vi "power.vi"(0 "Channel Index":i32, 5 "Clear PCM Sticky Faults":bool, 7 "Tare PDP Currents":bool, 9 "Clear PDP Sticky Faults":bool, 11 "Reset PDP Energy":bool) -> (4 "roboRIO":T4, 6 "Rail Voltages":T3, 8 "PCM":T2, 10 "PDP":T1, 13 "Channel Content":string, 15 "OutputsEnabled?":bool)   [LabVIEW 2014]
uses:
  Type Defs/power data.ctl
  <vilib>/Rock Robotics/Network Tables/NT Read String Array.vi
  <vilib>/Rock Robotics/Network Tables/NT Write Boolean Array.vi
  <vilib>/Rock Robotics/Network Tables/NT Read Boolean Array.vi
  <vilib>/Rock Robotics/Network Tables/NT Read Numeric Array.vi
  <vilib>/Rock Robotics/Network Tables/NT Read String.vi
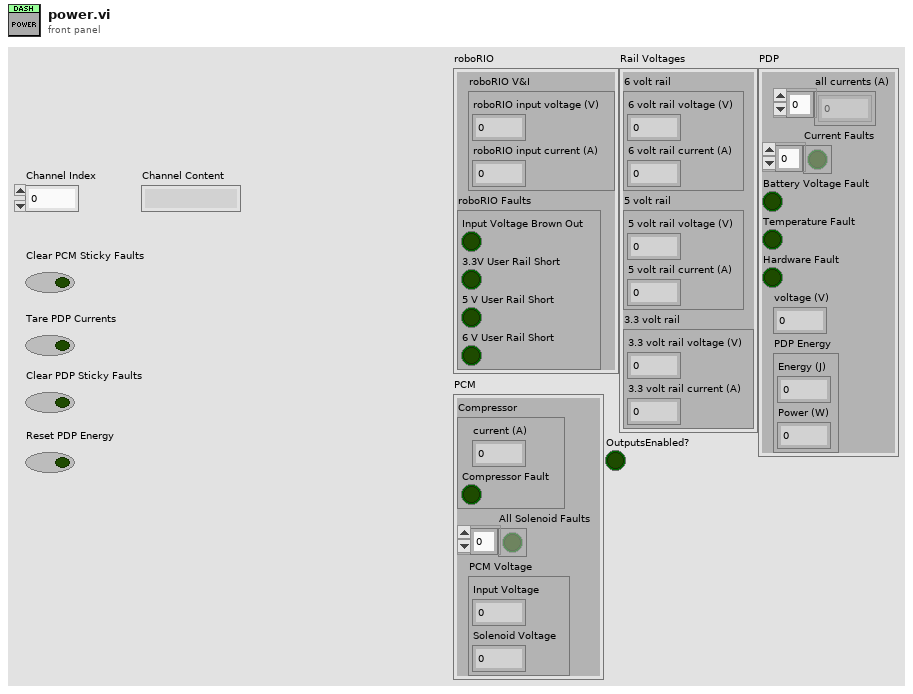
[diagram p1: front panel]
types:
  T1 = cluster{"all currents (A)":dbl[], "Current Faults":bool[], "Battery Voltage Fault":bool, "Temperature Fault":bool, "Hardware Fault":bool, "voltage (V)":dbl, "PDP Energy":cluster{"Energy (J)":dbl, "Power (W)":dbl}}
  T2 = cluster{"Compressor":cluster{"current (A)":dbl, "Compressor Fault":bool}, "All Solenoid Faults":bool[], "PCM Voltage":cluster{"Input Voltage":dbl, "Solenoid Voltage":dbl}}
  T3 = cluster{"6 volt rail":cluster{"6 volt rail voltage (V)":dbl, "6 volt rail current (A)":dbl}, "5 volt rail":cluster{"5 volt rail voltage (V)":dbl, "5 volt rail current (A)":dbl}, "3.3 volt rail":cluster{"3.3 volt rail voltage (V)":dbl, "3.3 volt rail current (A)":dbl}}
  T4 = cluster{"roboRIO V&I":cluster{"roboRIO input voltage (V)":dbl, "roboRIO input current (A)":dbl}, "roboRIO Faults":cluster{"Input Voltage Brown Out":bool, "3.3V User Rail Short":bool, "5 V User Rail Short":bool, "6 V User Rail Short":bool}}
  T5 = typedef "power data.ctl" = cluster{"roboRIO":cluster{"roboRIO V&I":cluster{"roboRIO input voltage (V)":dbl, "roboRIO input current (A)":dbl}, "roboRIO Faults":cluster{"Input Voltage Brown Out":bool, "3.3V User Rail Short":bool, "5 V User Rail Short":bool, "6 V User Rail Short":bool}}, "Rail Voltages":cluster{"6 volt rail":cluster{"6 volt rail voltage (V)":dbl, "6 volt rail current (A)":dbl}, "5 volt rail":cluster{"5 volt rail voltage (V)":dbl, "5 volt rail current (A)":dbl}, "3.3 volt rail":cluster{"3.3 volt rail voltage (V)":dbl, "3.3 volt rail current (A)":dbl}}, "PCM":cluster{"Compressor":cluster{"current (A)":dbl, "Compressor Fault":bool}, "All Solenoid Faults":bool[], "PCM Voltage":cluster{"Input Voltage":dbl, "Solenoid Voltage":dbl}}, "PDP":cluster{"all currents (A)":dbl[], "Current Faults":bool[], "Battery Voltage Fault":bool, "Temperature Fault":bool, "Hardware Fault":bool, "voltage (V)":dbl, "PDP Energy":cluster{"Energy (J)":dbl, "Power (W)":dbl}}, "OutputsEnabled?":bool}
  T6 = cluster{"current (A)":dbl, "Compressor Fault":bool}
  T7 = cluster{"Input Voltage":dbl, "Solenoid Voltage":dbl}
  T8 = cluster{"3.3 volt rail voltage (V)":dbl, "3.3 volt rail current (A)":dbl}
  T9 = cluster{"5 volt rail voltage (V)":dbl, "5 volt rail current (A)":dbl}
  T10 = cluster{"6 volt rail voltage (V)":dbl, "6 volt rail current (A)":dbl}
  T11 = cluster{"Input Voltage Brown Out":bool, "3.3V User Rail Short":bool, "5 V User Rail Short":bool, "6 V User Rail Short":bool}
  T12 = cluster{"roboRIO input voltage (V)":dbl, "roboRIO input current (A)":dbl}
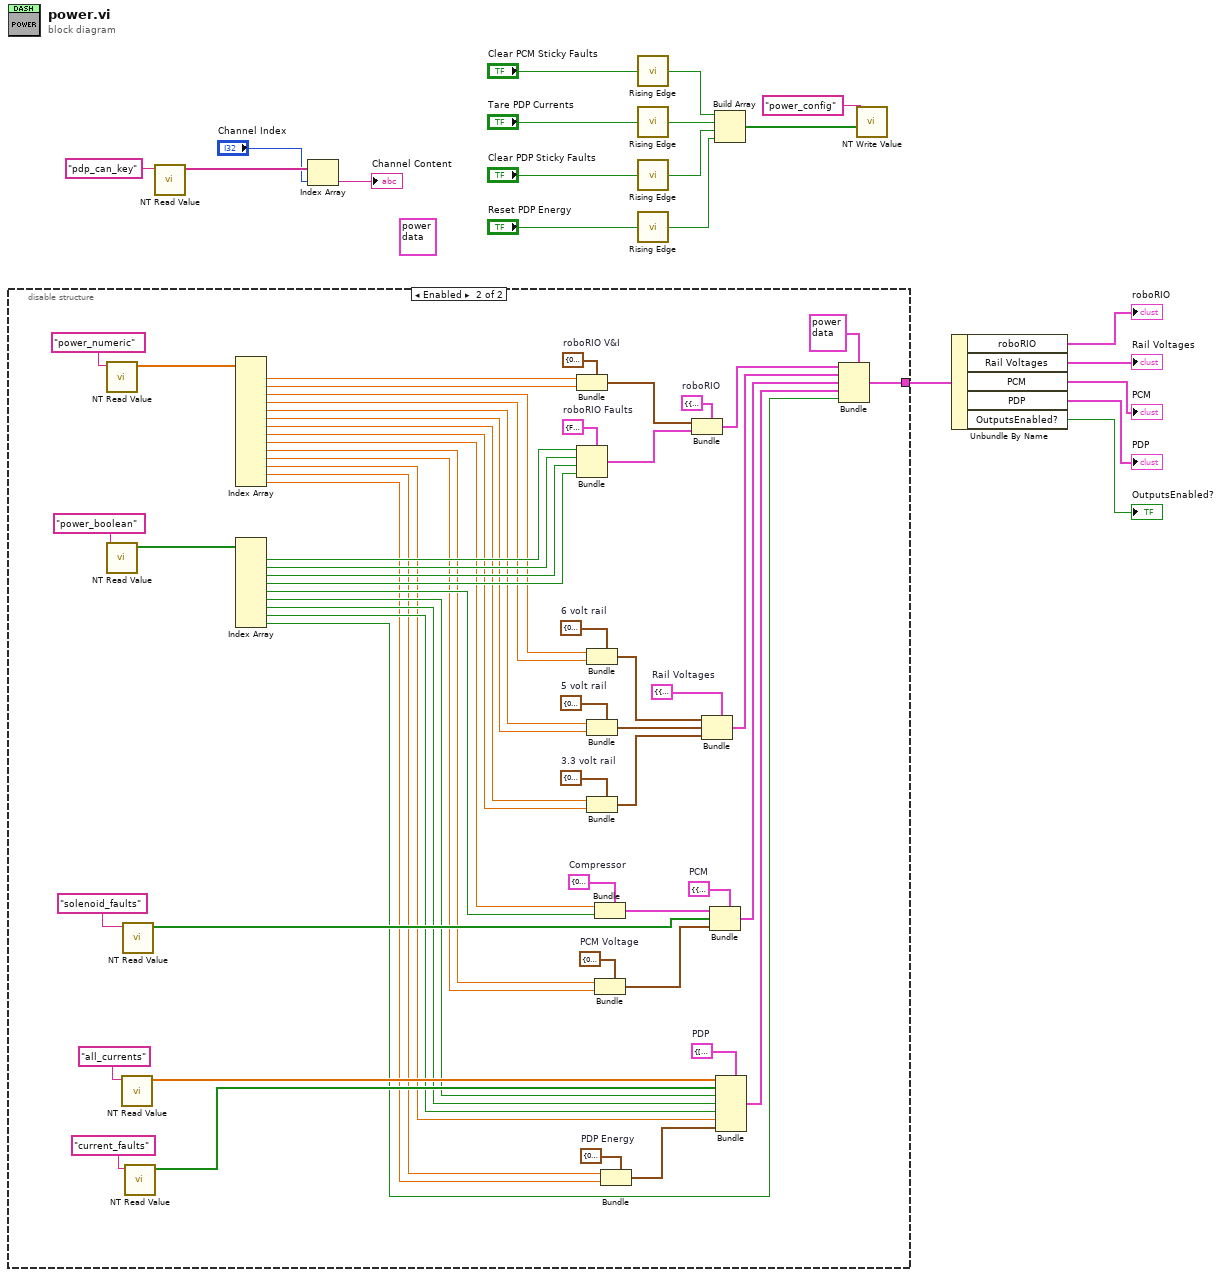
[diagram p0: block diagram]
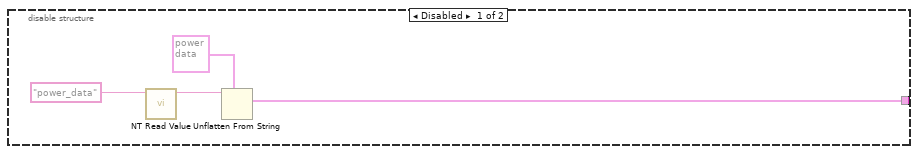
[diagram p2: hidden frame]
diagram:
  (unwired) T5 {"roboRIO"={"roboRIO V&I"={"roboRIO input voltage (V)"=0.0, "roboRIO input current (A)"=0.0}, "roboRIO Faults"={"Input Voltage Brown Out"=FALSE, "3.3V User Rail Short"=FALSE, "5 V User Rail Short"=FALSE, "6 V User Rail Short"=FALSE}}, "Rail Voltages"={"6 volt rail"={"6 volt rail voltage (V)"=0.0, "6 volt rail current (A)"=0.0}, "5 volt rail"={"5 volt rail voltage (V)"=0.0, "5 volt rail current (A)"=0.0}, "3.3 volt rail"={"3.3 volt rail voltage (V)"=0.0, "3.3 volt rail current (A)"=0.0}}, "PCM"={"Compressor"={"current (A)"=0.0, "Compressor Fault"=FALSE}, "All Solenoid Faults"=[], "PCM Voltage"={"Input Voltage"=0.0, "Solenoid Voltage"=0.0}}, "PDP"={"all currents (A)"=[], "Current Faults"=[], "Battery Voltage Fault"=FALSE, "Temperature Fault"=FALSE, "Hardware Fault"=FALSE, "voltage (V)"=0.0, "PDP Energy"={"Energy (J)"=0.0, "Power (W)"=0.0}}, "OutputsEnabled?"=FALSE} ("Power Data")
  n1 = disable-structure shown="Enabled" {
    disable-tunnel: [w21 w54] -> w20
    frame Disabled {
      n2 = call-poly <vilib>:"NT Read Value.vi"("Name"="power_data") -> ("String"=w23:string)  [unwired: 9 in, 1 out]
      n3 = Unflatten From String(type=T5 {"roboRIO"={"roboRIO V&I"={"roboRIO input voltage (V)"=0.0, "roboRIO input current (A)"=0.0}, "roboRIO Faults"={"Input Voltage Brown Out"=FALSE, "3.3V User Rail Short"=FALSE, "5 V User Rail Short"=FALSE, "6 V User Rail Short"=FALSE}}, "Rail Voltages"={"6 volt rail"={"6 volt rail voltage (V)"=0.0, "6 volt rail current (A)"=0.0}, "5 volt rail"={"5 volt rail voltage (V)"=0.0, "5 volt rail current (A)"=0.0}, "3.3 volt rail"={"3.3 volt rail voltage (V)"=0.0, "3.3 volt rail current (A)"=0.0}}, "PCM"={"Compressor"={"current (A)"=0.0, "Compressor Fault"=FALSE}, "All Solenoid Faults"=[], "PCM Voltage"={"Input Voltage"=0.0, "Solenoid Voltage"=0.0}}, "PDP"={"all currents (A)"=[], "Current Faults"=[], "Battery Voltage Fault"=FALSE, "Temperature Fault"=FALSE, "Hardware Fault"=FALSE, "voltage (V)"=0.0, "PDP Energy"={"Energy (J)"=0.0, "Power (W)"=0.0}}, "OutputsEnabled?"=FALSE} ("Power Data"), binary string=w23) -> (value=w21:T5)  [unwired: 3 in, 2 out]
    }
    frame Enabled {
      w38 = cluster{"Energy (J)":dbl, "Power (W)":dbl} {"Energy (J)"=0.0, "Power (W)"=0.0}  # PDP Energy
      w37 = T1 {"all currents (A)"=[], "Current Faults"=[], "Battery Voltage Fault"=FALSE, "Temperature Fault"=FALSE, "Hardware Fault"=FALSE, "voltage (V)"=0.0, "PDP Energy"={"Energy (J)"=0.0, "Power (W)"=0.0}}  # PDP
      w48 = T2 {"Compressor"={"current (A)"=0.0, "Compressor Fault"=FALSE}, "All Solenoid Faults"=[], "PCM Voltage"={"Input Voltage"=0.0, "Solenoid Voltage"=0.0}}  # PCM
      w49 = T6 {"current (A)"=0.0, "Compressor Fault"=FALSE}  # Compressor
      w50 = T7 {"Input Voltage"=0.0, "Solenoid Voltage"=0.0}  # PCM Voltage
      w65 = T3 {"6 volt rail"={"6 volt rail voltage (V)"=0.0, "6 volt rail current (A)"=0.0}, "5 volt rail"={"5 volt rail voltage (V)"=0.0, "5 volt rail current (A)"=0.0}, "3.3 volt rail"={"3.3 volt rail voltage (V)"=0.0, "3.3 volt rail current (A)"=0.0}}  # Rail Voltages
      w62 = T8 {"3.3 volt rail voltage (V)"=0.0, "3.3 volt rail current (A)"=0.0}  # 3.3 volt rail
      w63 = T9 {"5 volt rail voltage (V)"=0.0, "5 volt rail current (A)"=0.0}  # 5 volt rail
      w64 = T10 {"6 volt rail voltage (V)"=0.0, "6 volt rail current (A)"=0.0}  # 6 volt rail
      w80 = T11 {"Input Voltage Brown Out"=FALSE, "3.3V User Rail Short"=FALSE, "5 V User Rail Short"=FALSE, "6 V User Rail Short"=FALSE}  # roboRIO Faults
      w79 = T12 {"roboRIO input voltage (V)"=0.0, "roboRIO input current (A)"=0.0}  # roboRIO V&I
      w81 = T4 {"roboRIO V&I"={"roboRIO input voltage (V)"=0.0, "roboRIO input current (A)"=0.0}, "roboRIO Faults"={"Input Voltage Brown Out"=FALSE, "3.3V User Rail Short"=FALSE, "5 V User Rail Short"=FALSE, "6 V User Rail Short"=FALSE}}  # roboRIO
      n4 = call-poly <vilib>:"NT Read Value.vi"("Name"="power_numeric") -> ("Numeric Array"=w76:dbl[])  [unwired: 9 in, 1 out]
      n5 = call-poly <vilib>:"NT Read Value.vi"("Name"="power_boolean") -> ("Boolean Array"=w75:bool[])  [unwired: 9 in, 1 out]
      n6 = call-poly <vilib>:"NT Read Value.vi"("Name"="all_currents") -> ("Numeric Array"=w35:dbl[])  [unwired: 9 in, 1 out]
      n7 = call-poly <vilib>:"NT Read Value.vi"("Name"="solenoid_faults") -> ("Boolean Array"=w46:bool[])  [unwired: 9 in, 1 out]
      n8 = call-poly <vilib>:"NT Read Value.vi"("Name"="current_faults") -> ("Boolean Array"=w33:bool[])  [unwired: 9 in, 1 out]
      n9 = Index Array(array=w76) -> (element #1=w74:dbl, element #2=w73:dbl, element #3=w61:dbl, element #4=w60:dbl, element #5=w59:dbl, element #6=w58:dbl, element #7=w57:dbl, element #8=w56:dbl, element #9=w45:dbl, element #10=w43:dbl, element #11=w42:dbl, element #12=w29:dbl, element #13=w28:dbl, element #14=w27:dbl)  [unwired: 14 in]
      n10 = Index Array(array=w75) -> (element #1=w72:bool, element #2=w71:bool, element #3=w70:bool, element #4=w69:bool, element #5=w44:bool, element #6=w32:bool, element #7=w31:bool, element #8=w30:bool, element #9=w25:bool)  [unwired: 9 in]
      n11 = Bundle(cluster=w79, "roboRIO input voltage (V)"=w74, "roboRIO input current (A)"=w73) -> (w82:T12)
      n12 = Bundle(cluster=w80, "Input Voltage Brown Out"=w72, "3.3V User Rail Short"=w71, "5 V User Rail Short"=w70, "6 V User Rail Short"=w69) -> (w83:T11)
      n13 = Bundle(cluster=w64, "6 volt rail voltage (V)"=w61, "6 volt rail current (A)"=w60) -> (w66:T10)
      n14 = Bundle(cluster=w63, "5 volt rail voltage (V)"=w59, "5 volt rail current (A)"=w58) -> (w67:T9)
      n15 = Bundle(cluster=w62, "3.3 volt rail voltage (V)"=w57, "3.3 volt rail current (A)"=w56) -> (w68:T8)
      n16 = Bundle(cluster=w49, "current (A)"=w45, "Compressor Fault"=w44) -> (w51:T6)
      n17 = Bundle(cluster=w50, "Input Voltage"=w43, "Solenoid Voltage"=w42) -> (w52:T7)
      n18 = Bundle(cluster=w38, "Energy (J)"=w28, "Power (W)"=w27) -> (w39:cluster{"Energy (J)":dbl, "Power (W)":dbl})
      n19 = Bundle(cluster=w81, "roboRIO V&I"=w82, "roboRIO Faults"=w83) -> (w53:T4)
      n20 = Bundle(cluster=w65, "6 volt rail"=w66, "5 volt rail"=w67, "3.3 volt rail"=w68) -> (w41:T3)
      n21 = Bundle(cluster=w48, "Compressor"=w51, "All Solenoid Faults"=w46, "PCM Voltage"=w52) -> (w40:T2)
      n22 = Bundle(cluster=w37, "all currents (A)"=w35, "Current Faults"=w33, "Battery Voltage Fault"=w32, "Temperature Fault"=w31, "Hardware Fault"=w30, "voltage (V)"=w29, "PDP Energy"=w39) -> (w26:T1)
      n23 = Bundle(cluster=T5 {"roboRIO"={"roboRIO V&I"={"roboRIO input voltage (V)"=0.0, "roboRIO input current (A)"=0.0}, "roboRIO Faults"={"Input Voltage Brown Out"=FALSE, "3.3V User Rail Short"=FALSE, "5 V User Rail Short"=FALSE, "6 V User Rail Short"=FALSE}}, "Rail Voltages"={"6 volt rail"={"6 volt rail voltage (V)"=0.0, "6 volt rail current (A)"=0.0}, "5 volt rail"={"5 volt rail voltage (V)"=0.0, "5 volt rail current (A)"=0.0}, "3.3 volt rail"={"3.3 volt rail voltage (V)"=0.0, "3.3 volt rail current (A)"=0.0}}, "PCM"={"Compressor"={"current (A)"=0.0, "Compressor Fault"=FALSE}, "All Solenoid Faults"=[], "PCM Voltage"={"Input Voltage"=0.0, "Solenoid Voltage"=0.0}}, "PDP"={"all currents (A)"=[], "Current Faults"=[], "Battery Voltage Fault"=FALSE, "Temperature Fault"=FALSE, "Hardware Fault"=FALSE, "voltage (V)"=0.0, "PDP Energy"={"Energy (J)"=0.0, "Power (W)"=0.0}}, "OutputsEnabled?"=FALSE} ("Power Data"), "roboRIO"=w53, "Rail Voltages"=w41, "PCM"=w40, "PDP"=w26, "OutputsEnabled?"=w25) -> (w54:T5)
    }
  }
  n24 = call-poly <vilib>:"NT Read Value.vi"("Name"="pdp_can_key") -> ("String Array"=w14:string[])  [unwired: 9 in, 1 out]
  n25 = Index Array(array=w14, index="Channel Index") -> (element=→"Channel Content":string)
  n26 = call "Rising Edge.vi"("Input"="Clear PCM Sticky Faults") -> ("Rising Edge"=w7:bool)
  n27 = call "Rising Edge.vi"("Input"="Tare PDP Currents") -> ("Rising Edge"=w1:bool)
  n28 = call "Rising Edge.vi"("Input"="Clear PDP Sticky Faults") -> ("Rising Edge"=w3:bool)
  n29 = call "Rising Edge.vi"("Input"="Reset PDP Energy") -> ("Rising Edge"=w5:bool)
  n30 = Build Array(w7, w1, w3, w5) -> (w8:bool[])
  n31 = call-poly <vilib>:"NT Write Value.vi"("Boolean Array"=w8, "Name"="power_config") -> ()  [unwired: 9 in, 1 out]
  n32 = Unbundle By Name(w20) -> ("roboRIO"=→"roboRIO":T4, "Rail Voltages"=→"Rail Voltages":T3, "PCM"=→"PCM":T2, "PDP"=→"PDP":T1, "OutputsEnabled?"=→"OutputsEnabled?":bool)
